vi "IMAQdx_Flea3_get_attrib.vi"(4 "error in":errorcluster, 6 "attribute":string, 7 "IMAQdx in":T1) -> (0 "error out":errorcluster, 2 "attrib out":variant, 3 "IMAQdx out":T1)   [LabVIEW 2012]
uses:
  <vilib>/userdefined/High Color/IMAQdx.ctl
  <resource>/objmgr/imaqdx.rc
panel:
  out "error out 2":errorcluster
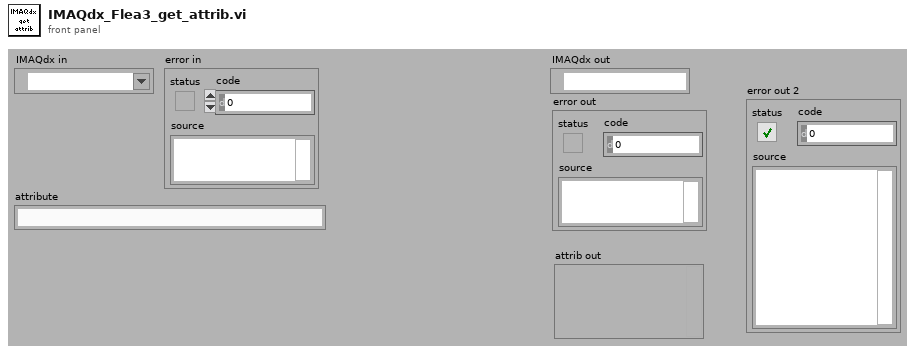
[diagram p1: front panel]
types:
  T1 = typedef "IMAQdx.ctl" = refnum<k21>
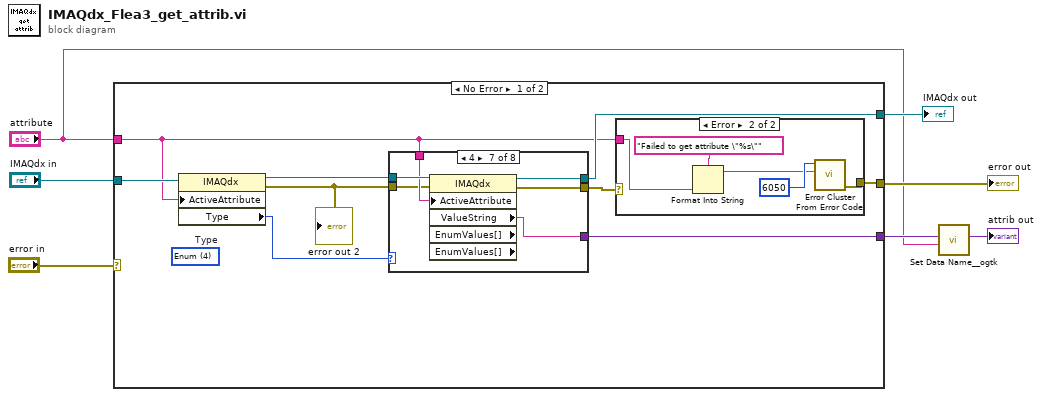
[diagram p0: block diagram]
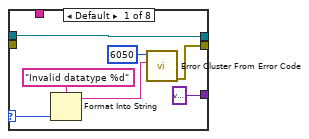
[diagram p3: hidden frame]
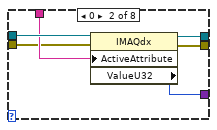
[diagram p4: hidden frame]
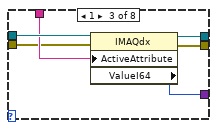
[diagram p5: hidden frame]
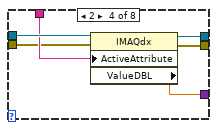
[diagram p6: hidden frame]
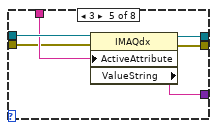
[diagram p7: hidden frame]
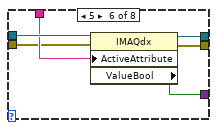
[diagram p8: hidden frame]
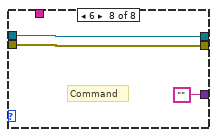
[diagram p9: hidden frame]
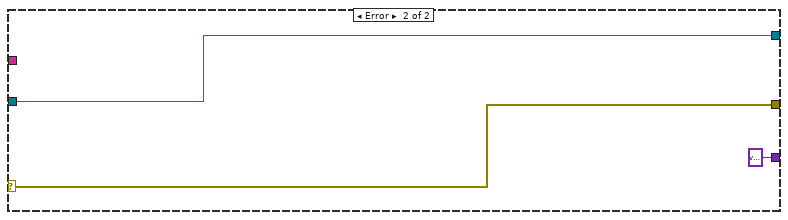
[diagram p10: hidden frame]
diagram:
  n1 = case shown="No Error" "error in" {
    selector: "error in" -> [_ w70]
    tunnel: [w16 w69] -> w7
    tunnel: "IMAQdx in" -> [w12 w69]
    tunnel: "attribute" -> [w9 _]
    tunnel: [w14 w70] -> w5
    tunnel: [w13 variant ("Variant")] -> w3
    frame No Error {
      (unwired) u32 4 items=["U32", "I64", "DBL", "String", "Enum", "Bool", "Command"]  # Type
      n2 = property class="IMAQdx"(reference=w12, "ActiveAttribute"=w9) -> (reference out=w10:T1, error out=w11:errorcluster, "Type"=w8:u32)  [unwired: 1 in]
      "error out 2" <- w11
      n3 = case shown="4" w8 {
        selector: w8 -> [w27 _ _ _ _ _ _ _]
        tunnel: [w28 w34 w40 w46 w52 w58 w64 w67] -> w16
        tunnel: w10 -> [w28 w33 w39 w45 w51 w57 w63 w67]
        tunnel: w9 -> [_ w32 w38 w44 w50 w56 w62 _]
        tunnel: [w24 w31 w37 w43 w49 w55 w61 w66] -> w15
        tunnel: [variant ("Variant") w30 w36 w42 w48 w54 w59 ""] -> w13
        tunnel: w11 -> [_ w29 w35 w41 w47 w53 w60 w66]
        frame Default {
          n4 = Format Into String(format string="Invalid datatype %d", w27) -> (resulting string=w23:string)  [unwired: 2 in, 1 out]
          n5 = call <vilib>:"Error Cluster From Error Code.vi"("error message (\"\")"=w23, "error code (0)"=6050) -> ("error out"=w24:errorcluster)  [unwired: 7 in]
        }
        frame 0 {
          n6 = property class="IMAQdx"(reference=w33, error in=w29, "ActiveAttribute"=w32) -> (reference out=w34:T1, error out=w31:errorcluster, "ValueU32"=w30:u32)
        }
        frame 1 {
          n7 = property class="IMAQdx"(reference=w39, error in=w35, "ActiveAttribute"=w38) -> (reference out=w40:T1, error out=w37:errorcluster, "ValueI64"=w36:i64)
        }
        frame 2 {
          n8 = property class="IMAQdx"(reference=w45, error in=w41, "ActiveAttribute"=w44) -> (reference out=w46:T1, error out=w43:errorcluster, "ValueDBL"=w42:dbl)
        }
        frame 3 {
          n9 = property class="IMAQdx"(reference=w51, error in=w47, "ActiveAttribute"=w50) -> (reference out=w52:T1, error out=w49:errorcluster, "ValueString"=w48:string)
        }
        frame 5 {
          n10 = property class="IMAQdx"(reference=w57, error in=w53, "ActiveAttribute"=w56) -> (reference out=w58:T1, error out=w55:errorcluster, "ValueBool"=w54:bool)
        }
        frame 4 {
          n11 = property class="IMAQdx" props=["ActiveAttribute", "ValueString", "EnumValues[]", "EnumValues[]"](reference=w63, error in=w60, "ActiveAttribute"=w62) -> (reference out=w64:T1, error out=w61:errorcluster, "ValueString"=w59:string)  [unwired: 2 out]
        }
        frame 6 {
          # "Command"
        }
      }
      n12 = case shown="Error" w15 {
        tunnel: w9 -> [_ w18]
        tunnel: [_ w17] -> w14
        frame No Error {
        }
        frame Error {
          n13 = Format Into String(format string="Failed to get attribute \"%s\"", w18) -> (resulting string=w19:string)  [unwired: 2 in, 1 out]
          n14 = call <vilib>:"Error Cluster From Error Code.vi"("error message (\"\")"=w19, "error code (0)"=6050) -> ("error out"=w17:errorcluster)  [unwired: 7 in]
        }
      }
    }
    frame Error {
    }
  }
  "IMAQdx out" <- w7
  "error out" <- w5
  n15 = call <userlib>:"Set Data Name__ogtk.vi"("Data Name"="attribute", "Data"=w3) -> ("Renamed Data"=→"attrib out":variant)  [unwired: 8 in, 1 out]
